vi "log_PerisPump.vi"(2 "read string":string, 3 "write string":string) -> (0 "PerisPump_read":string[](array[string]), 1 "PerisPump_write":string[](array[string]))   [LabVIEW 2023]
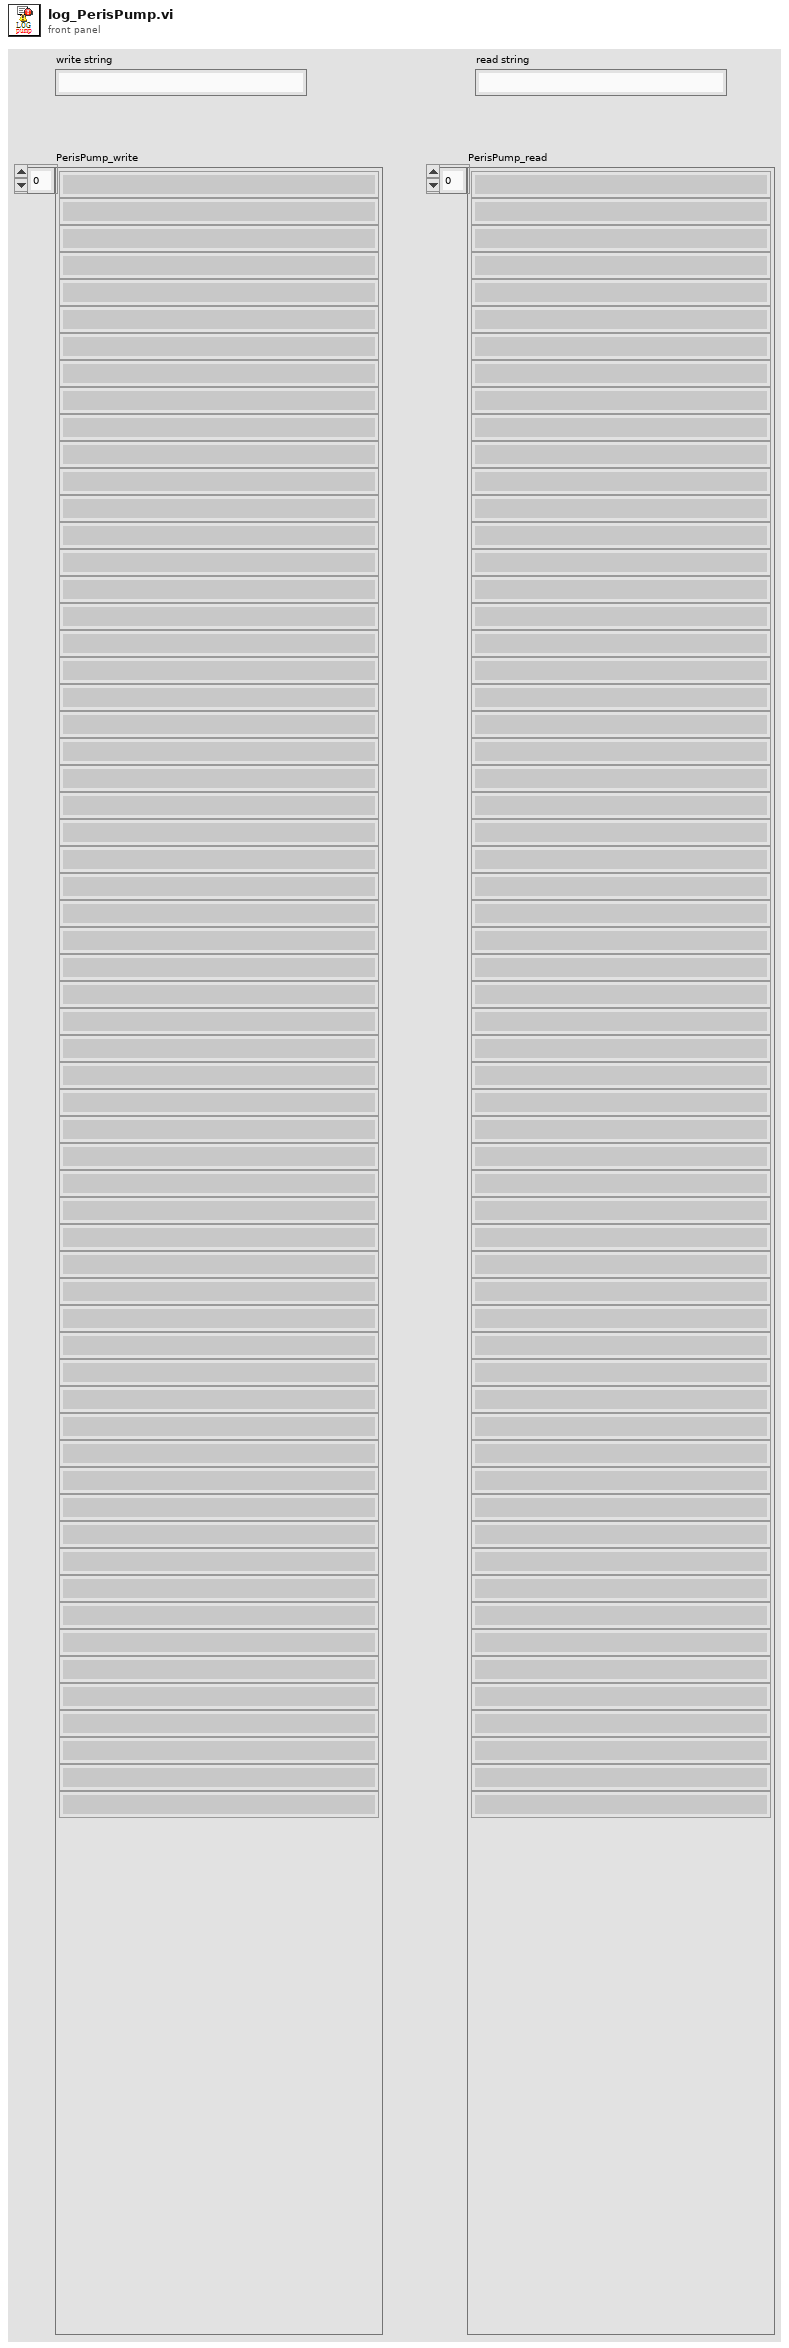
[diagram p1: front panel]
types:
  T1 = enum16{"open", "replace", "create", "open or create", "replace or create", "replace or create with confirmation"}
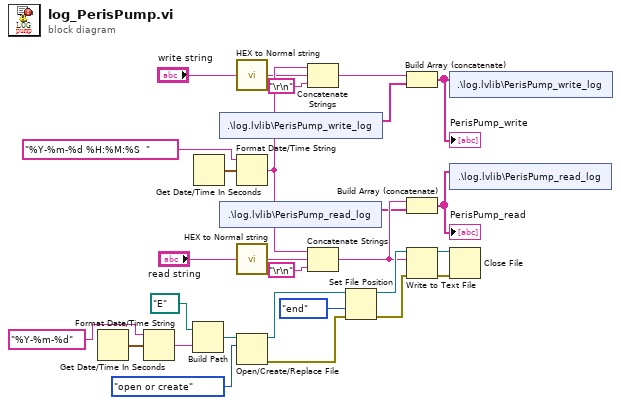
[diagram p0: block diagram]
diagram:
  n1 = Get Date/Time In Seconds() -> (seconds since 1Jan1904=w25:timestamp)
  n2 = Format Date/Time String(time format string (%c)="%Y-%m-%d", seconds (now)=w25) -> (date/time string=w26:string)  [unwired: 1 in]
  n3 = Build Path(base path=path "E:/", name or relative path=w26) -> (appended path=w18:path)
  n4 = Get Date/Time In Seconds() -> (seconds since 1Jan1904=w28:timestamp)
  n5 = shared-variable ".\\log.lvlib\\PerisPump_write_log"() -> (w5:string[])  [unwired: 1 in, 1 out]
  n6 = shared-variable ".\\log.lvlib\\PerisPump_read_log"() -> (w10:string[])  [unwired: 1 in, 1 out]
  n7 = call "HEX to Normal string.vi"("input hex string"="write string") -> ("String"=w6:string)
  n8 = Format Date/Time String(time format string (%c)="%Y-%m-%d %H:%M:%S  ", seconds (now)=w28) -> (date/time string=w7:string)  [unwired: 1 in]
  n9 = call "HEX to Normal string.vi"("input hex string"="read string") -> ("String"=w11:string)
  n10 = Open/Create/Replace File(file path (use dialog)=w18, operation (0:open)=T1."open or create") -> (refnum out=w21:refnum<file>, error out=w22:errorcluster)  [unwired: 4 in, 1 out]
  n11 = Concatenate Strings(w7, w6, "\r\n") -> (w4:string)
  n12 = Concatenate Strings(w7, w11, "\r\n") -> (w13:string)
  n13 = Set File Position(refnum=w21, from (0:start)=enum16{"start", "end", "current"}."end", error in=w22) -> (refnum out=w23:refnum<file>, error out=w24:errorcluster)  [unwired: 1 in]
  n14 = Build Array (concatenate)(w4, w5) -> (w3:string[])
  "PerisPump_write" <- w3
  n15 = Build Array (concatenate)(w13, w10) -> (w9:string[])
  "PerisPump_read" <- w9
  n16 = Write to Text File(file (use dialog)=w23, text=w13, error in=w24) -> (refnum out=w20:refnum<file>, error out=w19:errorcluster)  [unwired: 1 in, 1 out]
  n17 = shared-variable ".\\log.lvlib\\PerisPump_write_log"(w3) -> ()  [unwired: 1 in, 1 out]
  n18 = shared-variable ".\\log.lvlib\\PerisPump_read_log"(w9) -> ()  [unwired: 1 in, 1 out]
  n19 = Close File(refnum=w20, error in=w19) -> ()  [unwired: 2 out]
